vi "03 - Demonstration - High Throughput Transport Mechanism.vi"() -> ()   [LabVIEW 2012]
uses:
  <vilib>/picture/picture.llb/imagedata.ctl
panel:
  out "Small Events/sec":dbl caption="Events Throughput" format="%_4f events/sec"
  out "Picture 2":picture
  out "Picture 1":picture
  out "MB/sec":dbl caption="Data Throughput" format="%.2f MB/sec (x2)"
  in  "stop":bool
  out "Color Box 2":u32(colorbox)
  out "Color Box 1":u32(colorbox)
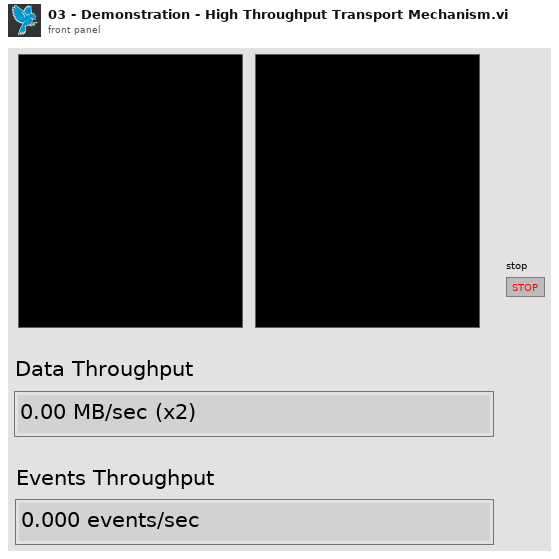
[diagram p1: front panel]
types:
  T1 = typedef "imagedata.ctl" = cluster{"image type":i32, "image depth":i32, "image":u8[], "mask":u8[], "colors":u32[], "Rectangle":cluster{"left":i16, "top":i16, "right":i16, "bottom":i16}}
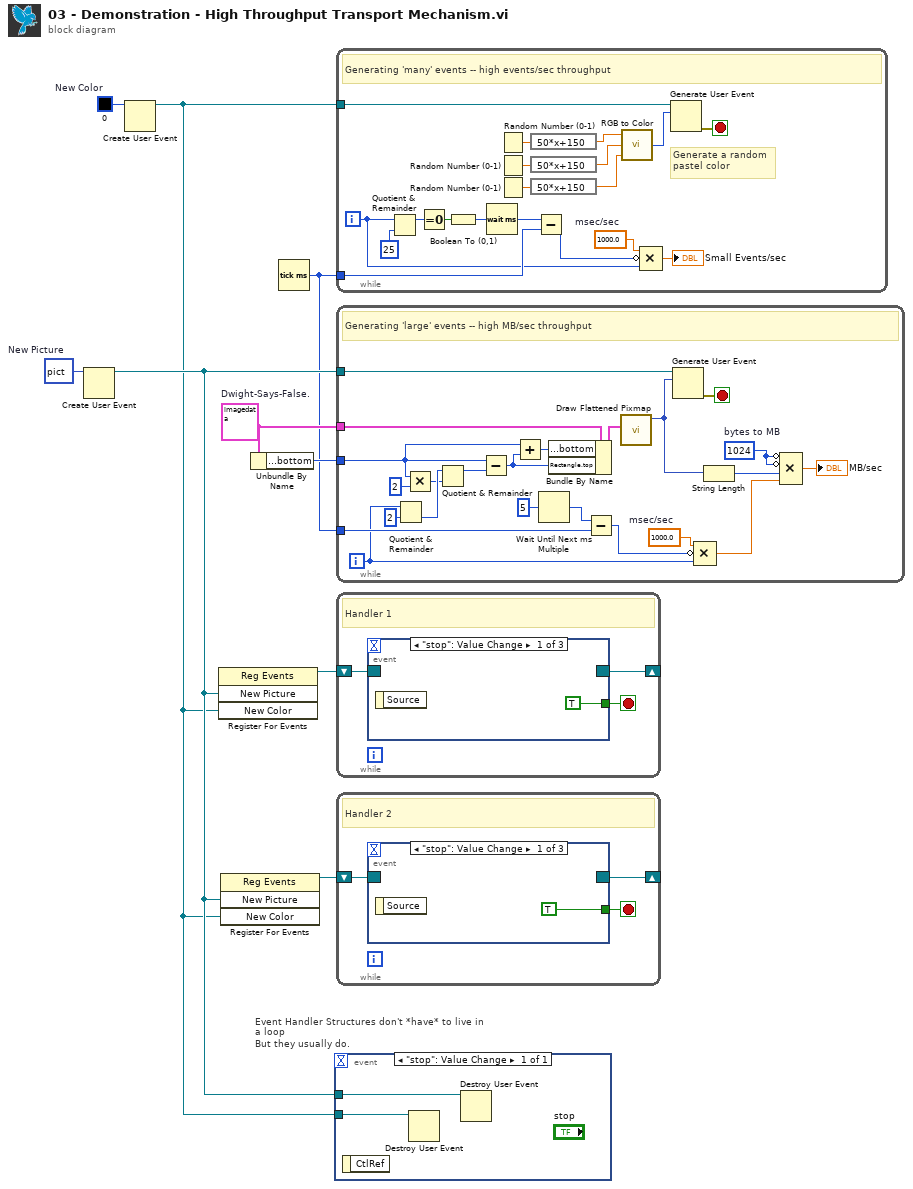
[diagram p0: block diagram]
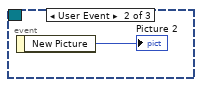
[diagram p2: hidden frame]
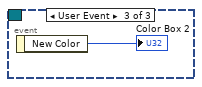
[diagram p3: hidden frame]
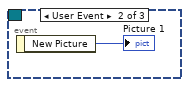
[diagram p4: hidden frame]
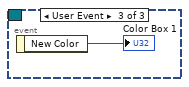
[diagram p5: hidden frame]
diagram:
  w4 = u32 0  # New Color
  w6 = T1 {"image type"=0, "image depth"=32, "image"=array[234768 elements], "mask"=array[7504 elements], "colors"=[], "Rectangle"={"left"=0, "top"=0, "right"=219, "bottom"=268}}  # Dwight-Says-False.
  w7 = picture data[5B]  # New Picture
  n1 = Create User Event(user event datatype=w7) -> (user event=w3:refnum<user-event>)  [unwired: 1 in, 1 out]
  n2 = Create User Event(user event datatype=w4) -> (user event=w2:refnum<user-event>)  [unwired: 1 in, 1 out]
  n3 = register-events(w3, w2) -> (reference out=w9:refnum<event-registration>)  [unwired: 2 in, 1 out]
  n4 = register-events(w3, w2) -> (reference out=w8:refnum<event-registration>)  [unwired: 2 in, 1 out]
  n5 = Unbundle By Name(w6) -> ("Rectangle.bottom"=w5:i16)
  n6 = Tick Count (ms)() -> (millisecond timer value=w1:u32)
  n7 = event "Event Handler Structures don't *have* to live in a loop\nBut they usually do." shown="[0] \"stop\": Value Change" {
    selector: _ -> [_]
    dyn-events: _ -> [_]
    timeout: _ -> [_]
    tunnel: w3 -> [w10]
    tunnel: w2 -> [w11]
    event "stop": Value Change {
      n8 = event-data() -> ()  [unwired: 1 in, 1 out]
      n9 = Destroy User Event(user event=w11) -> ()  [unwired: 1 in, 1 out]
      n10 = Destroy User Event(user event=w10) -> ()  [unwired: 1 in, 1 out]
    }
  }
  n11 = while {
    tunnel: w2 -> [w30]
    tunnel: w1 -> [w23]
    i -> [w20]
    stop <- w28 stop-if-true
    w22 = 1000.0  # msec/sec
    # "Generate a random\npastel color"
    # "Generating 'many' events -- high events/sec throughput"
    n12 = Quotient & Remainder(x=w20, y=25) -> (x-y*floor(x/y)=w26:i32)  [unwired: 1 out]
    n13 = Equal To 0?(x=w26) -> (x = 0?=w25:bool)
    n14 = Boolean To (0,1)(Boolean=w25) -> (0, 1=w18:i16)
    n15 = Wait (ms)(milliseconds to wait=w18) -> (millisecond timer value=w24:u32)
    n16 = Random Number (0-1)() -> (number: 0 to 1=w17:dbl)
    n17 = Random Number (0-1)() -> (number: 0 to 1=w15:dbl)
    n18 = Random Number (0-1)() -> (number: 0 to 1=w14:dbl)
    n19 = expression code="50*x+150"(w17) -> (w16:dbl)
    n20 = expression code="50*x+150"(w15) -> (w12:dbl)
    n21 = expression code="50*x+150"(w14) -> (w13:dbl)
    n22 = Subtract(x=w24, y=w23) -> (x-y=w21:u32)
    n23 = call <vilib>:"RGB to Color.vi"("B"=w13, "G"=w12, "R"=w16) -> ("Color"=w29:u32)
    n24 = Compound Arithmetic op=MULTIPLY(w22, invert w21, w20) -> (→"Small Events/sec":dbl)
    n25 = Generate User Event(user event=w30, event data cluster=w29) -> (error out=w28:errorcluster)  [unwired: 1 in, 1 out]
  }
  n26 = while {
    tunnel: w3 -> [w52]
    tunnel: w1 -> [w51]
    tunnel: w6 -> [w42]
    tunnel: w5 -> [w31]
    i -> [w39]
    stop <- w36 stop-if-true
    w45 = 1024  # bytes to MB
    w49 = 1000.0  # msec/sec
    # "Generating 'large' events -- high MB/sec throughput"
    n27 = Quotient & Remainder(x=w39, y=2) -> (floor(x/y)=w41:i32)  [unwired: 1 out]
    n28 = Multiply(x=w31, y=i16 2) -> (x*y=w32:i16)
    n29 = Quotient & Remainder(x=w41, y=w32) -> (x-y*floor(x/y)=w35:i32)  [unwired: 1 out]
    n30 = Subtract(x=w31, y=w35) -> (x-y=w34:i32)
    n31 = Add(x=w31, y=w34) -> (x+y=w37:i32)
    n32 = Wait Until Next ms Multiple(millisecond multiple=u32 5 ("milliseconds to wait")) -> (millisecond timer value=w38:u32)
    n33 = Bundle By Name(cluster=w42, "Rectangle.bottom"=w37, "Rectangle.top"=w34) -> (w43:T1)
    n34 = Subtract(x=w38, y=w51) -> (x-y=w50:u32)
    n35 = call <vilib>:"Draw Flattened Pixmap.vi"("image data"=w43) -> ("new picture"=w44:picture)  [unwired: 8 in]
    n36 = Generate User Event(user event=w52, event data cluster=w44) -> (error out=w36:errorcluster)  [unwired: 1 in, 1 out]
    n37 = Compound Arithmetic op=MULTIPLY(w49, invert w50, w39) -> (w47:dbl)
    n38 = String Length(string=w44) -> (length=w48:i32)
    n39 = Compound Arithmetic op=MULTIPLY(invert w45, invert w45, w48, w47) -> (→"MB/sec":dbl)
  }
  n40 = while {
    shift-right: [w55] -> _
    shift-left: w9 -> [w56]
    stop <- w54 stop-if-true
    # "Handler 1"
    n41 = event shown="[0] \"stop\": Value Change" {
      selector: w56 -> [_ _ _]
      dyn-events: [_ _ _] -> w55
      timeout: _ -> [_ _ _]
      tunnel: [TRUE _ _] -> w54
      event "stop": Value Change {
        n42 = event-data() -> ()  [unwired: 1 in, 1 out]
      }
      event User Event {
        n43 = event-data() -> ("New Picture"=→"Picture 1":picture)  [unwired: 1 in]
      }
      event User Event {
        n44 = event-data() -> ("New Color"=→"Color Box 1":u32)  [unwired: 1 in]
      }
    }
  }
  n45 = while {
    shift-right: [w61] -> _
    shift-left: w8 -> [w62]
    stop <- w60 stop-if-true
    # "Handler 2"
    n46 = event shown="[0] \"stop\": Value Change" {
      selector: w62 -> [_ _ _]
      dyn-events: [_ _ _] -> w61
      timeout: _ -> [_ _ _]
      tunnel: [TRUE _ _] -> w60
      event "stop": Value Change {
        n47 = event-data() -> ()  [unwired: 1 in, 1 out]
      }
      event User Event {
        n48 = event-data() -> ("New Picture"=→"Picture 2":picture)  [unwired: 1 in]
      }
      event User Event {
        n49 = event-data() -> ("New Color"=→"Color Box 2":u32)  [unwired: 1 in]
      }
    }
  }
